vi "lockin_Vsg_multichannel.vi"(10 "Comments":string="Vbg=-0.4V\nsweep Vsg: -100mV to 25mV, 0.5mV steps\nxxxsweep B : 14T --> -14T, 0.0028 A/s\n\n300ms wait between gate values\ntime constant =1E-2 s\norder=2\n\nlockin settings: \n1: 1, current, 0mV AC, 13 Hz, 50kOhm shunt resistor, gain=100\n2: 2, voltage, gain=100\n3: 3, voltage, gain=100\n4: 5, voltage, gain=100\n5: 7, current, 100uV AC, -350uV DC, 13 Hz, 50kOhm shunt resistor, gain=100\n6: 9, voltage, gain=100\n", 11 "ITX folder":string="18 - sweep Vsg, small amp") -> ()   [LabVIEW 2013]
uses:
  cryogenic ltd/state machine/state machine/Cryogeni Global 1.vi
  <userlib>/Levylab/PPMS VI/SubVI/ITX_Global.vi
  Labview_Local/Lockin-4461_Multiple Inputs and Outputs_KH Folder/P/users1/Joe/Lockin-4461_3.0 4461-4462 Multichannel Folder/DAQ-Lockin-SubVI/Lock-in Globles Multiple Inputs and Outputs.vi
panel:
  in  "Tab Control":enum32{"Sweep BG", "lockin/SG Control", "Data"}(tab)=enum."lockin/SG Control"
  in  "Channels: AO":T1={"AO amp (V)"=[0.0, 0.0, 0.0, 0.0, 0.0001, 0.0, 0.0, 0.0], "AO DC (V)"=[0.0, 0.0, 0.0, 0.0, -0.00035, 0.0, 0.0, 0.0], "AO f (Hz)"=[13.0, 13.0, 13.0, 13.0, 13.0, 13.0, 13.0, 13.0], "AO phi (deg)"=[0.0, 0.0, 0.0, 0.0, 0.0, 0.0, 0.0, 0.0], "function"=[enum."Sine Wave", enum."Sine Wave", enum."Sine Wave", enum."Sine Wave", enum."Sine Wave", enum."Sine Wave", enum."Sine Wave", enum."Sine Wave"]} {"AO DC (V)" format="%#_6p"; "AO amp (V)" format="%#_6p"}
  in  "Vmax (end)":dbl=0.075 format="%#_3p"
  in  "Vmin (start)":dbl=-0.1 format="%#_3p"
  in  "dV":dbl=0.001 format="%#_3p"
  out "T (mK)":dbl=14.454279
  in  "wait between Vsgs":u32=300
  in  "Initial wait":u32=10000
  in  "# of lockins":i32=6
  in  "\"channel\"":i32=6
  in  "Physical Channel":tag="PXI1Slot8/ao1"
  in  "T=sg\nF=bg":bool=TRUE
  in  "cycles (1,2,...)":i32=1 min=1 step=1
  in  "phase":dbl
  out "ramp rate":dbl=0.0214 format="%#_13g"
  out "Field":dbl=13.9996 format="%#_13g"
  in  "function (ramp)":enum16{"Ramp", "Triangle", "Sine"}(ring)
  in  "x":dbl
  out "Lockins":cluster{"Y":dbl[], "Y":dbl[]}[](graph)
  # "Vsg start = Vmin + X*B\nVsg end = Vsg start + Vmax\nMAKE X=0 IF YOU WANT TO\nSWEEP THE REGULAR WAY"
  # "0"
  # "1"
  # "2"
  # "3"
  # "4"
  # "5"
  # "6"
  # "7"
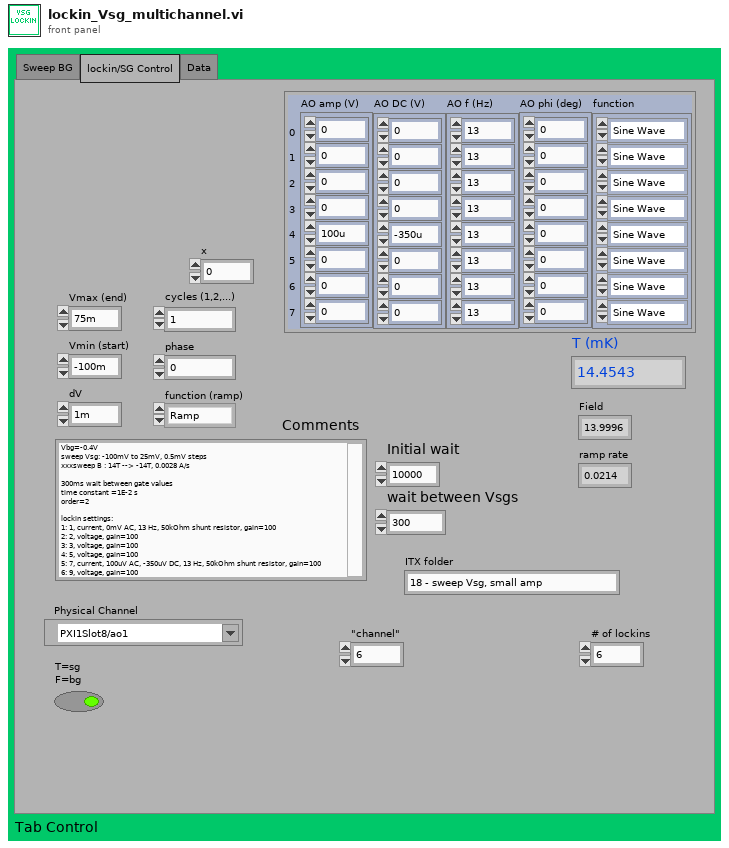
[diagram p1: front panel]
types:
  T1 = cluster{"AO amp (V)":dbl[], "AO DC (V)":dbl[], "AO f (Hz)":dbl[], "AO phi (deg)":dbl[], "function":enum16{"Sine Wave", "Triangle Wave", "Square Wave", "Sawtooth Wave"}[]}
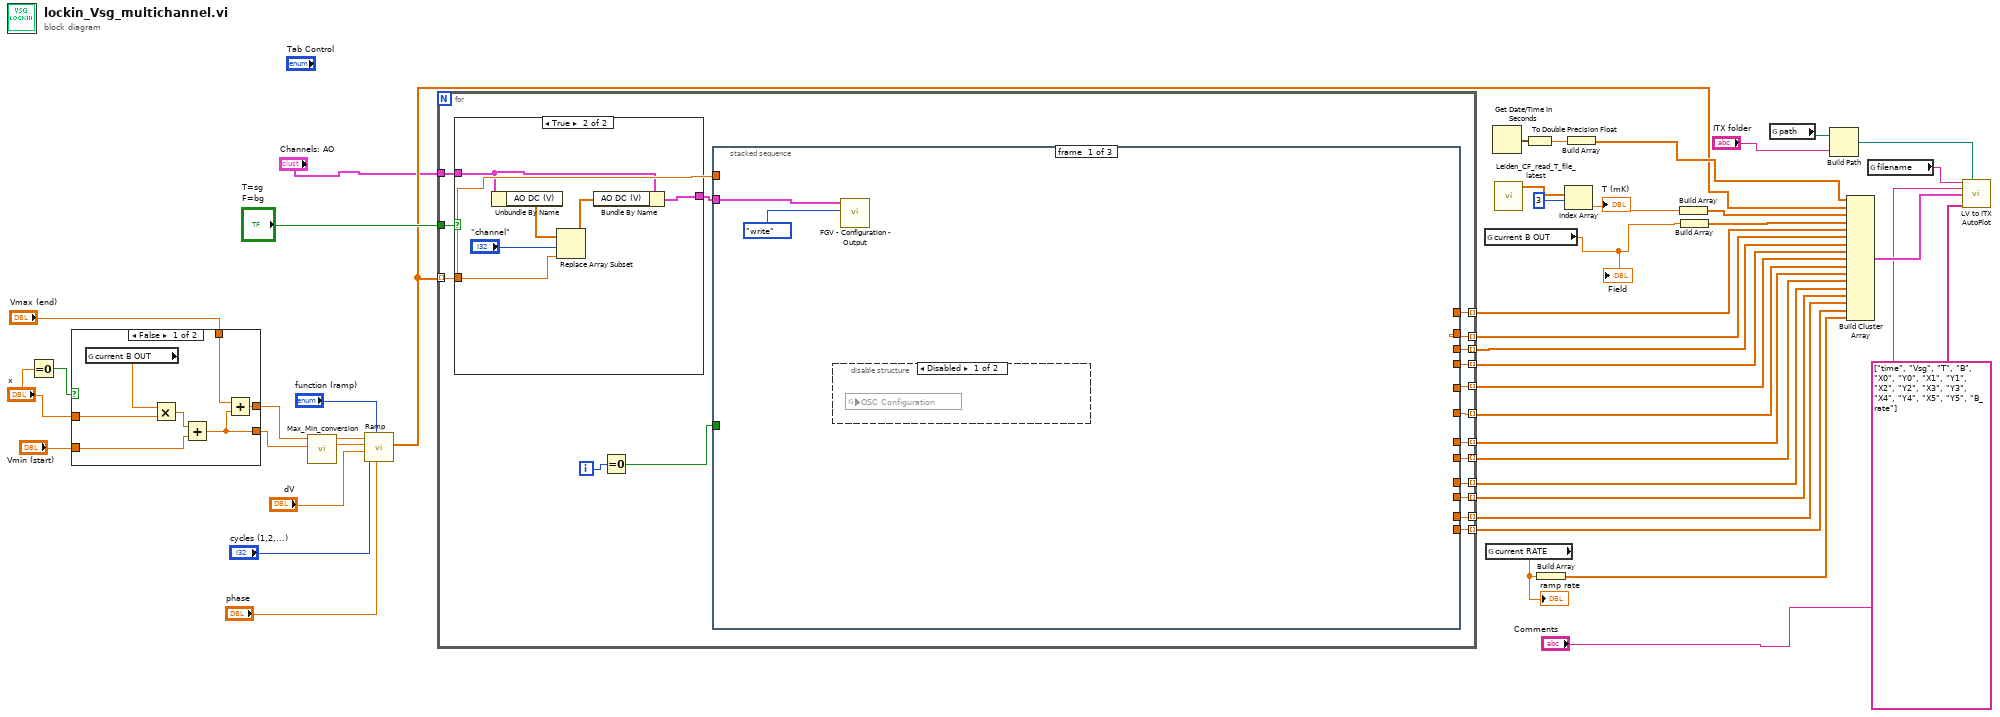
[diagram p0: block diagram]
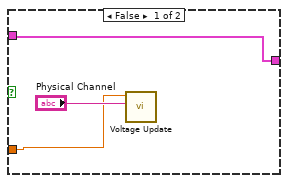
[diagram p3: hidden frame]
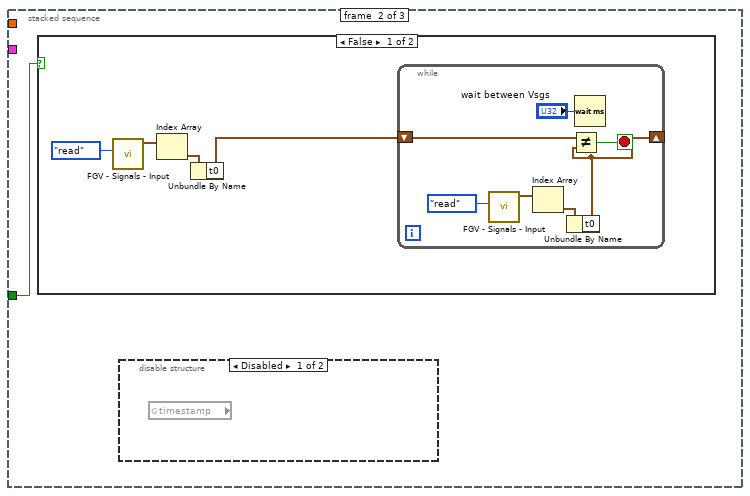
[diagram p5: hidden frame]
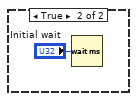
[diagram p7: hidden frame]
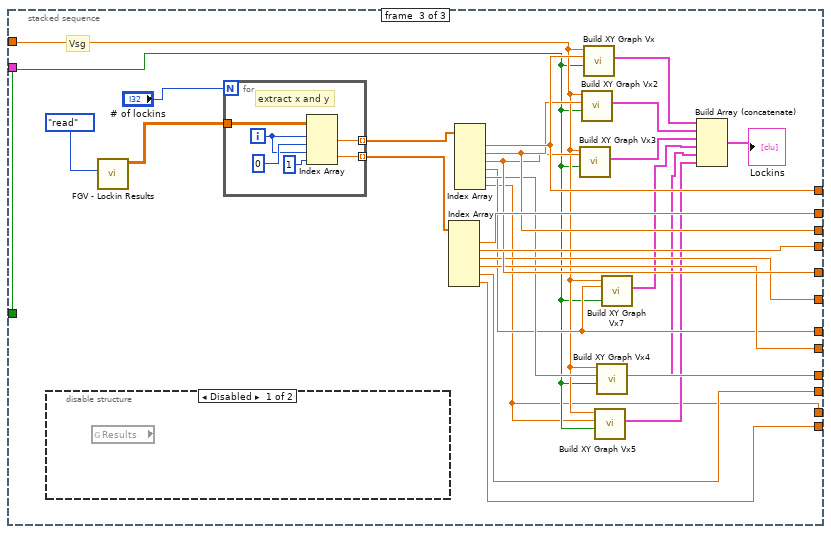
[diagram p8: hidden frame]
diagram:
  n1 = Equal To 0?(x="x") -> (x = 0?=w2:bool)
  n2 = case shown="False" w2 {
    tunnel: "Vmin (start)" -> [w50 w53]
    tunnel: [w49 w53] -> w6
    tunnel: [w48 w54] -> w5
    tunnel: "Vmax (end)" -> [w47 w54]
    tunnel: "x" -> [w46 _]
    frame False {
      n3 = global read "Cryogeni Global 1.vi" "current B OUT"() -> (w52:dbl)
      n4 = Multiply(x=w52, y=w46) -> (x*y=w51:dbl)
      n5 = Add(x=w51, y=w50) -> (x+y=w49:dbl)
      n6 = Add(x=w47, y=w49) -> (x+y=w48:dbl)
    }
    frame True {
    }
  }
  n7 = call <userlib>:"Max_Min_conversion.vi"("Min"=w6, "Max"=w5) -> ("offset"=w14:dbl, "Amplitude"=w15:dbl)  [unwired: 8 in]
  n8 = call <userlib>:"Ramp.vi"("phase"="phase", "function (ramp)"="function (ramp)", "cycles (1,2,...)"="cycles (1,2,...)", "step size"="dV", "offset"=w14, "amplitude"=w15) -> ("Waveform Graph"=w10:dbl[])  [unwired: 3 in, 2 out]
  n9 = for {
    tunnel: "Channels: AO" -> [w72]
    tunnel: w10 -> [w62] mode=indexing
    tunnel: [w68] -> w29 mode=indexing
    tunnel: [w67] -> w31 mode=indexing
    tunnel: [w66] -> w30 mode=indexing
    tunnel: [w65] -> w28 mode=indexing
    tunnel: [w64] -> w27 mode=indexing
    tunnel: [w63] -> w26 mode=indexing
    tunnel: [w61] -> w25 mode=indexing
    tunnel: [w60] -> w24 mode=indexing
    tunnel: [w59] -> w23 mode=indexing
    tunnel: [w58] -> w22 mode=indexing
    tunnel: [w57] -> w20 mode=indexing
    tunnel: [w56] -> w21 mode=indexing
    tunnel: "T=sg\nF=bg" -> [w55]
    i -> [w70]
    n10 = case shown="True" w55 {
      tunnel: w72 -> [w75 w81]
      tunnel: [w75 w76] -> w71
      tunnel: w62 -> [w73 w79]
      frame False {
        n11 = call <userlib>:"Voltage Update.vi"("Voltage Output"=w73, "Physical Channel"="Physical Channel") -> ()  [unwired: 7 in]
      }
      frame True {
        n12 = Unbundle By Name(w81) -> ("AO DC (V)"=w80:dbl[])
        n13 = Replace Array Subset(array=w80, new element=w79, index="\"channel\"") -> (w77:dbl[])
        n14 = Bundle By Name(cluster=w81, "AO DC (V)"=w77) -> (w76:T1)
      }
    }
    n15 = Equal To 0?(x=w70) -> (x = 0?=w69:bool)
    n16 = stacked-sequence {
      tunnel: w71 -> [w82 _ _]
      tunnel: w62 -> [_ _ w104]
      tunnel: w69 -> [_ w84 w103]
      tunnel: [_ _ w113] -> w68
      tunnel: [_ _ w115] -> w67
      tunnel: [_ _ w114] -> w66
      tunnel: [_ _ w112] -> w65
      tunnel: [_ _ w111] -> w64
      tunnel: [_ _ w110] -> w63
      tunnel: [_ _ w105] -> w61
      tunnel: [_ _ w109] -> w60
      tunnel: [_ _ w108] -> w59
      tunnel: [_ _ w107] -> w58
      tunnel: [_ _ w106] -> w57
      tunnel: [_ _ w99] -> w56
      frame #0 {
        n17 = disable-structure shown="Disabled" {
          frame Disabled {
            n18 = global read "Lock-in Globles Multiple Inputs and Outputs.vi" "OSC Configuration"() -> ()  [unwired: 1 in]
          }
          frame Enabled {
          }
        }
        n19 = call "FGV - Configuration - Output.vi"("Function"=enum16{"write", "read"}."write", "Channels: AO"=w82) -> ()  [unwired: 4 in, 2 out]
      }
      frame #1 {
        n20 = case shown="False" w84 {
          frame False {
            n21 = call "FGV - Signals - Input.vi"("Function"=enum16{"write", "read"}."read") -> ("input signal"=w87:waveform(dbl)[])  [unwired: 5 in, 1 out]
            n22 = Index Array(array=w87) -> (element=w86:waveform(dbl))  [unwired: 1 in]
            n23 = Unbundle By Name(w86) -> ("t0"=w85:timestamp)
            n24 = while {
              shift-right: [w90] -> _
              shift-left: w85 -> [w95]
              stop <- w94 stop-if-true
              n25 = call "FGV - Signals - Input.vi"("Function"=enum16{"write", "read"}."read") -> ("input signal"=w89:waveform(dbl)[])  [unwired: 5 in, 1 out]
              n26 = Index Array(array=w89) -> (element=w92:waveform(dbl))  [unwired: 1 in]
              n27 = Unbundle By Name(w92) -> ("t0"=w90:timestamp)
              n28 = Not Equal?(x=w95, y=w90) -> (x != y?=w94:bool)
              n29 = Wait (ms)(milliseconds to wait="wait between Vsgs") -> ()  [unwired: 1 out]
            }
          }
          frame True {
            n30 = Wait (ms)(milliseconds to wait="Initial wait") -> ()  [unwired: 1 out]
          }
        }
        n31 = disable-structure shown="Disabled" {
          frame Disabled {
            n32 = global read "Lock-in Globles Multiple Inputs and Outputs.vi" "timestamp"() -> ()  [unwired: 1 out]
          }
          frame Enabled {
          }
        }
      }
      frame #2 {
        # "Vsg"
        n33 = disable-structure shown="Disabled" {
          frame Disabled {
            n34 = global read "Lock-in Globles Multiple Inputs and Outputs.vi" "Results"() -> ()  [unwired: 1 out]
          }
          frame Enabled {
          }
        }
        n35 = call "FGV - Lockin Results.vi"("Function"=enum16{"write", "read"}."read") -> ("Input Signals"=w97:dbl[][])  [unwired: 5 in, 1 out]
        n36 = for {
          N: "# of lockins" -> [_]
          tunnel: w97 -> [w126]
          tunnel: [w124] -> w117 mode=indexing
          tunnel: [w123] -> w116 mode=indexing
          i -> [w125]
          # "extract x and y"
          n37 = Index Array(array=w126, index (row) #1=w125, index (col) #1=0 ("disabled index (col)"), index (row) #2=w125, index (col) #2=1 ("disabled index (col)")) -> (element #1=w124:dbl, element #2=w123:dbl)
        }
        n38 = Index Array(array=w116) -> (element #1=w114:dbl, element #2=w112:dbl, element #3=w110:dbl, element #4=w109:dbl, element #5=w107:dbl, element #6=w106:dbl)  [unwired: 6 in]
        n39 = Index Array(array=w117) -> (element #1=w115:dbl, element #2=w113:dbl, element #3=w111:dbl, element #4=w105:dbl, element #5=w108:dbl, element #6=w99:dbl)  [unwired: 6 in]
        n40 = call "Build XY Graph Vx3"("Reset"=w103, "Y Input"=w111, "X Input"=w104) -> ("XY Graph"=w120:cluster{"Y":dbl[], "Y":dbl[]}[])  [unwired: 2 in, 6 out]
        n41 = call "Build XY Graph Vx2"("Reset"=w103, "Y Input"=w113, "X Input"=w104) -> ("XY Graph"=w121:cluster{"Y":dbl[], "Y":dbl[]}[])  [unwired: 2 in, 6 out]
        n42 = call "Build XY Graph Vx"("Reset"=w103, "Y Input"=w115, "X Input"=w104) -> ("XY Graph"=w122:cluster{"Y":dbl[], "Y":dbl[]}[])  [unwired: 2 in, 6 out]
        n43 = call "Build XY Graph Vx5"("Reset"=w103, "Y Input"=w99, "X Input"=w104) -> ("XY Graph"=w100:cluster{"Y":dbl[], "Y":dbl[]}[])  [unwired: 2 in, 6 out]
        n44 = call "Build XY Graph Vx4"("Reset"=w103, "Y Input"=w108, "X Input"=w104) -> ("XY Graph"=w101:cluster{"Y":dbl[], "Y":dbl[]}[])  [unwired: 2 in, 6 out]
        n45 = call "Build XY Graph Vx7"("Reset"=w103, "Y Input"=w105, "X Input"=w104) -> ("XY Graph"=w102:cluster{"Y":dbl[], "Y":dbl[]}[])  [unwired: 2 in, 6 out]
        n46 = Build Array (concatenate)(w122, w121, w120, w102, w101, w100) -> (→"Lockins":cluster{"Y":dbl[], "Y":dbl[]}[])
      }
    }
  }
  n47 = global read "Cryogeni Global 1.vi" "current B OUT"() -> (w17:dbl)
  "Field" <- w17
  n48 = global read "Cryogeni Global 1.vi" "current RATE"() -> (w8:dbl)
  "ramp rate" <- w8
  n49 = Get Date/Time In Seconds() -> (seconds since 1Jan1904=w34:timestamp)
  n50 = call "Leiden_CF_read_T_file_latest.vi"() -> ("T array"=w36:dbl[])  [unwired: 11 in]
  n51 = To Double Precision Float(number=w34) -> (double precision float=w33:dbl)
  n52 = Build Array(w8) -> (w19:dbl[])
  n53 = Index Array(array=w36, index=3) -> (element=w39:dbl)
  "T (mK)" <- w39
  n54 = Build Array(w33) -> (w32:dbl[])
  n55 = Build Array(w39) -> (w38:dbl[])
  n56 = Build Array(w17) -> (w37:dbl[])
  n57 = global read "ITX_Global.vi" "path"() -> (w45:path)
  n58 = Build Path(base path=w45, name or relative path="ITX folder") -> (appended path=w44:path)
  n59 = Build Cluster Array(w32, w10, w38, w37, w31, w30, w29, w28, w27, w26, w25, w24, w23, w22, w21, w20, w19) -> (w42:cluster{"Waveform Graph":dbl[]}[])
  n60 = global read "ITX_Global.vi" "filename"() -> (w43:string)
  n61 = call <userlib>:"LV to ITX AutoPlot.vi"("filename"=w43, "path"=w44, "Notes"="Comments", "Data"=w42, "wavenames (.Vx, etc)"=string[] ["time", "Vsg", "T", "B", "X0", "Y0", "X1", "Y1", "X2", "Y2", "X3", "Y3", "X4", "Y4", "X5", "Y5", "B_rate"]) -> ()  [unwired: 10 in, 1 out]
